vi "Read Snake Head.vi"(8 "error in (no error)":errorcluster, 11 "Snake in":refnum<class "Snake.lvclass">) -> (0 "error out":errorcluster, 2 "position":cluster{"x":dbl, "y":dbl}, 3 "Snake out":refnum<class "Snake.lvclass">)   [LabVIEW 2021, in "Snake.lvclass"]
uses:
  Snake.lvclass
  C:/Users/poche/Programs/LabVIEW/imposible snake/GameEl_class/GameEl.lvclass
  GameEl_class/GameEl.lvclass/GameEl.ctl
  GameEl_class/Read position.vi
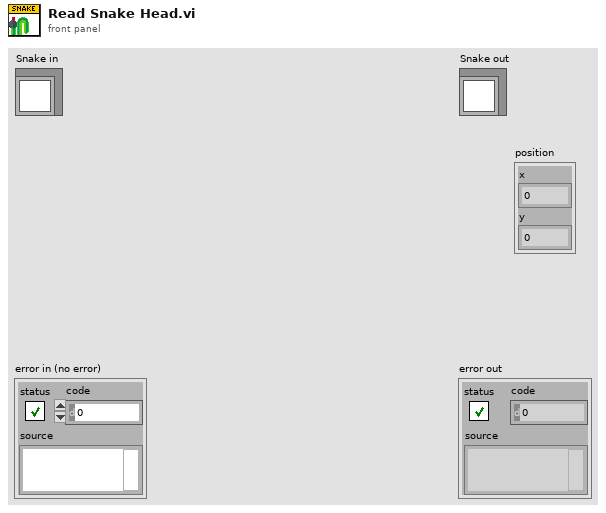
[diagram p1: front panel]
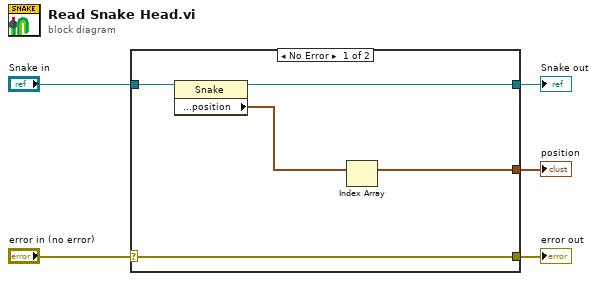
[diagram p0: block diagram]
diagram:
  n1 = case shown="No Error" "error in (no error)" {
    selector: "error in (no error)" -> [w10 w11]
    tunnel: [w10 w11] -> w4
    tunnel: [w7 w12] -> w2
    tunnel: "Snake in" -> [w9 w12]
    tunnel: [w8 _] -> w1
    frame No Error {
      n2 = property class="Snake"(reference=w9) -> (reference out=w7:refnum<class "Snake.lvclass">, "SubVIs:DataAccess:position"=w6:cluster{"x":dbl, "y":dbl}[])  [unwired: 1 in, 1 out]
      n3 = Index Array(array=w6) -> (element=w8:cluster{"x":dbl, "y":dbl})  [unwired: 1 in]
    }
    frame Error {
    }
  }
  "error out" <- w4
  "Snake out" <- w2
  "position" <- w1
